vi "MinDisplac(FinishP)1.vi"(4 "error IN":errorcluster, 7 "IN (X,Y,dX,dY)":dbl[][](array[numeric])) -> (0 "error OUT":errorcluster, 1 "Amount of finded Coinc":i32, 3 "OUT (X,Y,dX,dY) MINIMAL":dbl[][](array[numeric]))   [LabVIEW 2013]
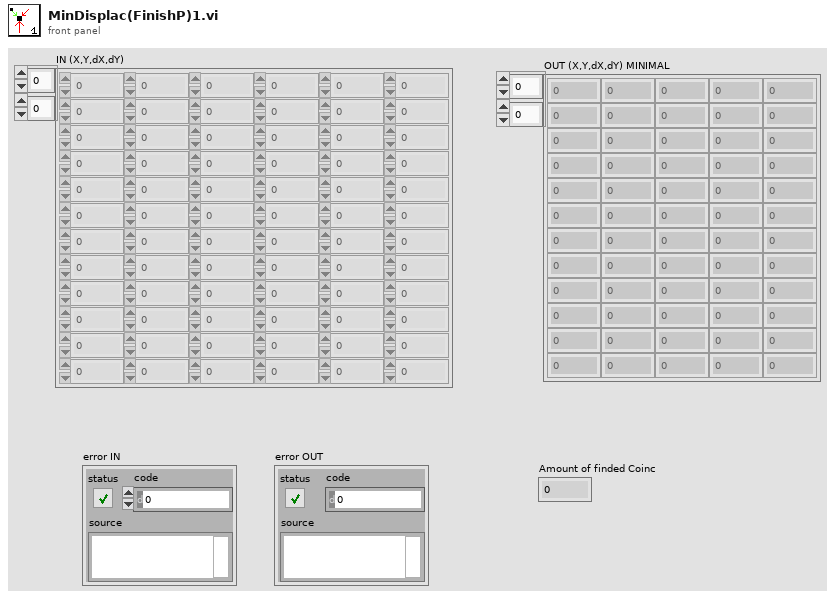
[diagram p1: front panel]
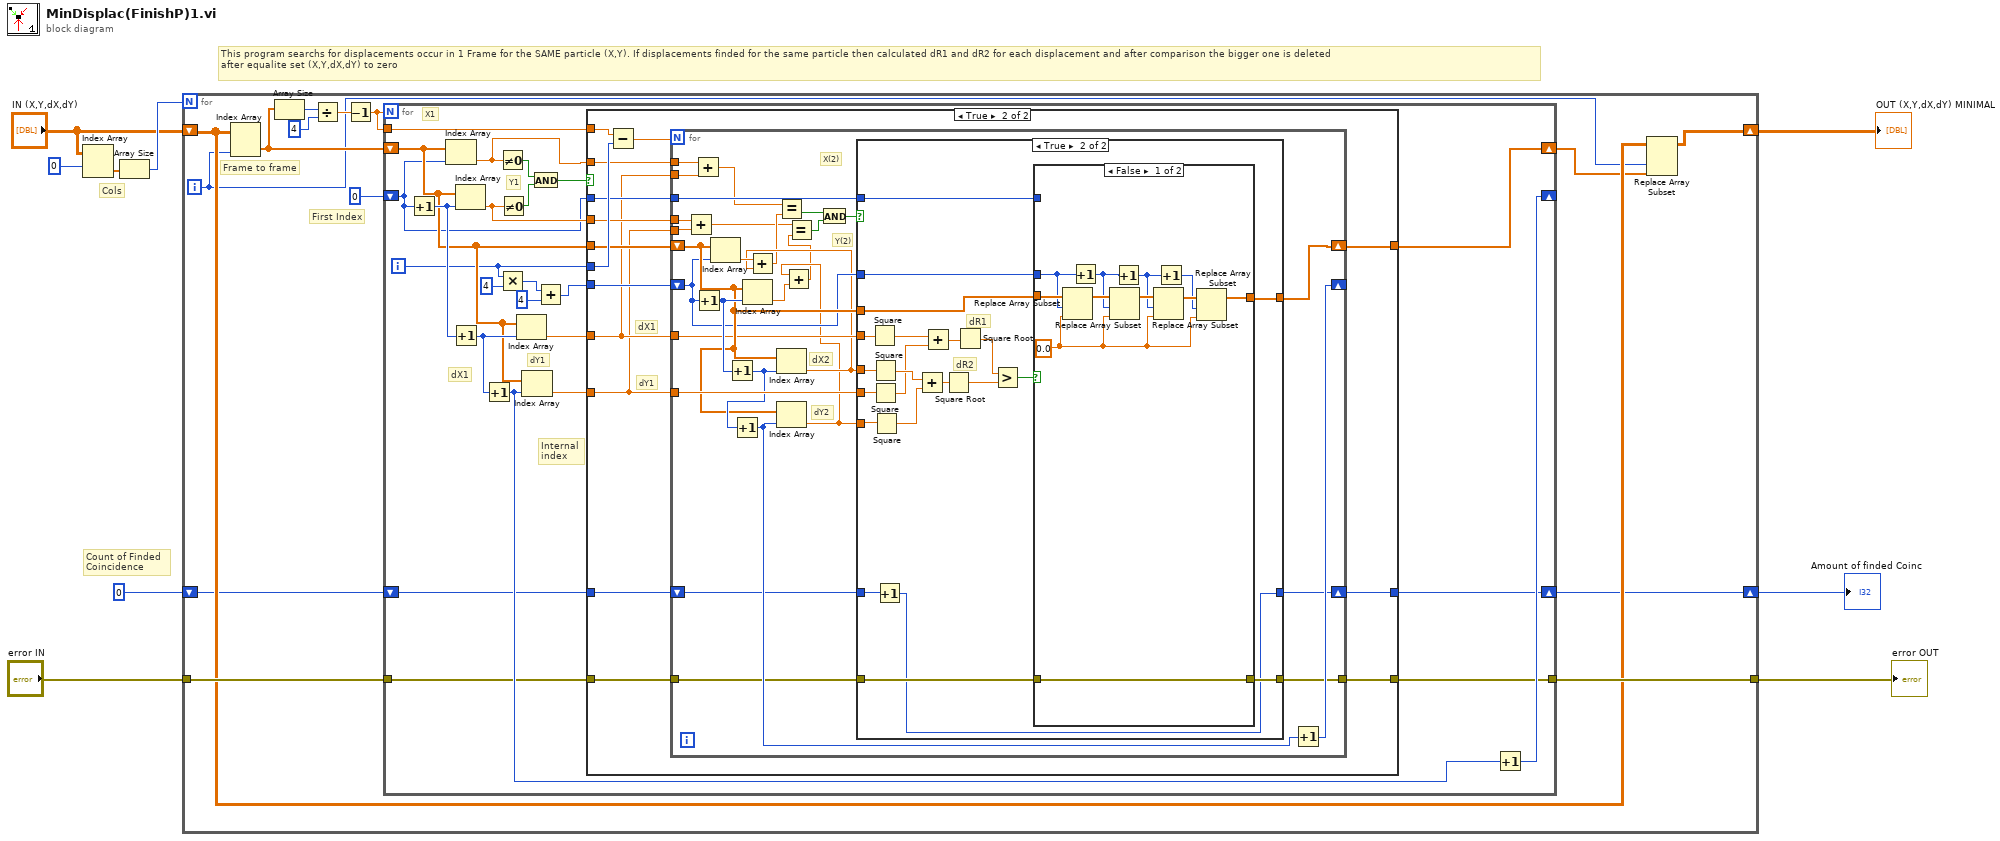
[diagram p0: block diagram]
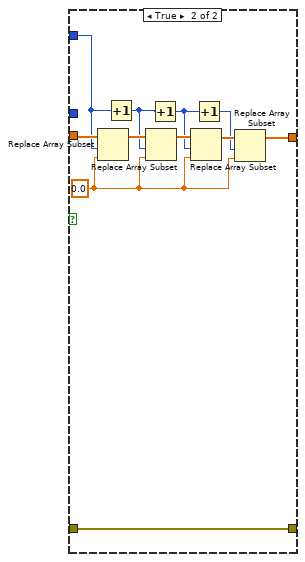
[diagram p4: hidden frame]
diagram:
  # "This program searchs for displacements occur in 1 Frame for the SAME particle (X,Y). If displacements finded for the same particle then calculated dR1 and dR2 for each displacement and after comparison the bigger one is deleted \nafter equalite set (X,Y,dX,dY) to zero"
  # "Count of Finded\nCoincidence"
  # "Cols"
  n1 = Index Array(array="IN (X,Y,dX,dY)", index (row)=0) -> (element=w8:dbl[])  [unwired: 1 in]
  n2 = Array Size(array=w8) -> (size(s)=w7:i32)
  n3 = for {
    N: w7 -> [_]
    shift-right: [w12] -> w3
    shift-left: "IN (X,Y,dX,dY)" -> [w15]
    tunnel: "error IN" -> [w17]
    tunnel: [w16] -> w4
    shift-right: [w10] -> w1
    shift-left: 0 -> [w11]
    i -> [w14]
    # "First Index"
    # "Frame to frame"
    n4 = Index Array(array=w15, index (col)=w14) -> (element=w22:dbl[])  [unwired: 1 in]
    n5 = Array Size(array=w22) -> (size(s)=w20:i32)
    n6 = Divide(x=w20, y=4) -> (x/y=w19:dbl)
    n7 = Decrement(x=w19) -> (x-1=w18:dbl)
    n8 = for {
      N: w18 -> [_]
      shift-right: [w27] -> w13
      shift-left: w22 -> [w39]
      shift-right: [w37] -> _
      shift-left: 0 -> [w29]
      tunnel: w18 -> [w44]
      tunnel: w17 -> [w28]
      tunnel: [w26] -> w16
      shift-right: [w24] -> w10
      shift-left: w11 -> [w25]
      i -> [w34]
      # "dX1"
      # "dY1"
      # "Internal \nindex"
      # "Y1"
      # "X1"
      n9 = Increment(x=w29) -> (x+1=w41:i32)
      n10 = Index Array(array=w39, index=w29) -> (element=w43:dbl)
      n11 = Increment(x=w41) -> (x+1=w40:i32)
      n12 = Index Array(array=w39, index=w41) -> (element=w42:dbl)
      n13 = Increment(x=w40) -> (x+1=w38:i32)
      n14 = Not Equal To 0?(x=w43) -> (x != 0?=w47:bool)
      n15 = Multiply(x=w34, y=4) -> (x*y=w32:i32)
      n16 = Not Equal To 0?(x=w42) -> (x != 0?=w46:bool)
      n17 = Index Array(array=w39, index=w40) -> (element=w36:dbl)
      n18 = Index Array(array=w39, index=w38) -> (element=w35:dbl)
      n19 = And(x=w47, y=w46) -> (x .and. y?=w45:bool)
      n20 = Add(x=w32, y=4) -> (x+y=w31:i32)
      n21 = case shown="True" w45 {
        tunnel: w44 -> [_ w65]
        tunnel: w34 -> [_ w64]
        tunnel: w43 -> [_ w61]
        tunnel: w42 -> [_ w60]
        tunnel: w39 -> [w50 w62]
        tunnel: [w50 w59] -> w27
        tunnel: w36 -> [_ w52]
        tunnel: w35 -> [_ w51]
        tunnel: w31 -> [_ w58]
        tunnel: w29 -> [_ w57]
        tunnel: w28 -> [w49 w56]
        tunnel: [w49 w55] -> w26
        tunnel: w25 -> [w48 w54]
        tunnel: [w48 w53] -> w24
        frame False {
        }
        frame True {
          # "dX1"
          # "dY1"
          n22 = Subtract(x=w65, y=w64) -> (x-y=w63:dbl)
          n23 = for {
            N: w63 -> [_]
            shift-right: [w84] -> w59
            shift-left: w62 -> [w86]
            tunnel: w61 -> [w78]
            tunnel: w60 -> [w75]
            shift-right: [w87] -> _
            shift-left: w58 -> [w83]
            tunnel: w52 -> [w77]
            tunnel: w51 -> [w91]
            tunnel: w57 -> [w85]
            tunnel: w56 -> [w82]
            tunnel: [w81] -> w55
            shift-right: [w79] -> w53
            shift-left: w54 -> [w80]
            tunnel: w52 -> [w76]
            tunnel: w51 -> [w74]
            # "Y(2)"
            # "X(2)"
            # "dY2"
            # "dX2"
            n24 = Add(x=w75, y=w74) -> (x+y=w69:dbl)
            n25 = Add(x=w78, y=w76) -> (x+y=w70:dbl)
            n26 = Increment(x=w83) -> (x+1=w90:i32)
            n27 = Index Array(array=w86, index=w83) -> (element=w73:dbl)
            n28 = Increment(x=w90) -> (x+1=w89:i32)
            n29 = Increment(x=w89) -> (x+1=w88:i32)
            n30 = Index Array(array=w86, index=w90) -> (element=w68:dbl)
            n31 = Index Array(array=w86, index=w89) -> (element=w72:dbl)
            n32 = Add(x=w73, y=w72) -> (x+y=w71:dbl)
            n33 = Equal?(x=w70, y=w71) -> (x = y?=w94:bool)
            n34 = Index Array(array=w86, index=w88) -> (element=w67:dbl)
            n35 = Add(x=w67, y=w68) -> (x+y=w66:dbl)
            n36 = Equal?(x=w69, y=w66) -> (x = y?=w93:bool)
            n37 = And(x=w94, y=w93) -> (x .and. y?=w92:bool)
            n38 = case shown="True" w92 {
              tunnel: w77 -> [_ w118]
              tunnel: w91 -> [_ w116]
              tunnel: w67 -> [_ w115]
              tunnel: w72 -> [_ w117]
              tunnel: w86 -> [w97 w107]
              tunnel: w85 -> [_ w106]
              tunnel: [w97 w105] -> w84
              tunnel: w83 -> [_ w104]
              tunnel: w82 -> [w96 w103]
              tunnel: [w96 w102] -> w81
              tunnel: w80 -> [w95 w101]
              tunnel: [w95 w100] -> w79
              frame False {
              }
              frame True {
                # "dR2"
                # "dR1"
                n39 = Square(x=w118) -> (x^2=w112:dbl)
                n40 = Square(x=w117) -> (x^2=w114:dbl)
                n41 = Square(x=w116) -> (x^2=w99:dbl)
                n42 = Square(x=w115) -> (x^2=w98:dbl)
                n43 = Increment(x=w101) -> (x+1=w100:i32)
                n44 = Add(x=w114, y=w98) -> (x+y=w113:dbl)
                n45 = Add(x=w112, y=w99) -> (x+y=w111:dbl)
                n46 = Square Root(x=w113) -> (sqrt(x)=w109:dbl)
                n47 = Square Root(x=w111) -> (sqrt(x)=w110:dbl)
                n48 = Greater?(x=w110, y=w109) -> (0:w108:bool)
                n49 = case shown="False" w108 {
                  tunnel: w107 -> [w122 w140]
                  tunnel: w106 -> [_ w138]
                  tunnel: [w120 w131] -> w105
                  tunnel: w104 -> [w121 _]
                  tunnel: [w119 w130] -> w102
                  tunnel: w103 -> [w119 w130]
                  frame False {
                    w126 = 0.0 ("new element/subarray")
                    n50 = Replace Array Subset(array=w122, new element=w126, index=w121) -> (w129:dbl[])
                    n51 = Increment(x=w121) -> (x+1=w125:i32)
                    n52 = Replace Array Subset(array=w129, new element=w126, index=w125) -> (w128:dbl[])
                    n53 = Increment(x=w125) -> (x+1=w124:i32)
                    n54 = Replace Array Subset(array=w128, new element=w126, index=w124) -> (w127:dbl[])
                    n55 = Increment(x=w124) -> (x+1=w123:i32)
                    n56 = Replace Array Subset(array=w127, new element=w126, index=w123) -> (w120:dbl[])
                  }
                  frame True {
                    w135 = 0.0 ("new element/subarray")
                    n57 = Replace Array Subset(array=w140, new element=w135, index=w138) -> (w139:dbl[])
                    n58 = Increment(x=w138) -> (x+1=w134:i32)
                    n59 = Replace Array Subset(array=w139, new element=w135, index=w134) -> (w137:dbl[])
                    n60 = Increment(x=w134) -> (x+1=w133:i32)
                    n61 = Replace Array Subset(array=w137, new element=w135, index=w133) -> (w136:dbl[])
                    n62 = Increment(x=w133) -> (x+1=w132:i32)
                    n63 = Replace Array Subset(array=w136, new element=w135, index=w132) -> (w131:dbl[])
                  }
                }
              }
            }
            n64 = Increment(x=w88) -> (x+1=w87:i32)
          }
        }
      }
      n65 = Increment(x=w38) -> (x+1=w37:i32)
    }
    n66 = Replace Array Subset(array=w15, new element=w13, index (col)=w14) -> (w12:dbl[][])  [unwired: 1 in]
  }
  "error OUT" <- w4
  "OUT (X,Y,dX,dY) MINIMAL" <- w3
  "Amount of finded Coinc" <- w1
